vi "Launch Handler.vi"(7 "App Refnum":refnum<vi>, 8 "User action":bool=TRUE, 9 "Open":bool=TRUE, 10 "Diagram":bool=TRUE, 11 "VI":string) -> ()   [LabVIEW 2020, in "Peek Window.lvlib"]
uses:
  Peek Window.lvlib
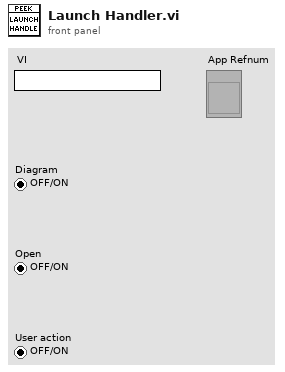
[diagram p1: front panel]
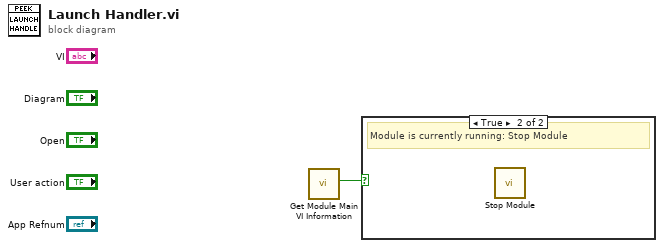
[diagram p0: block diagram]
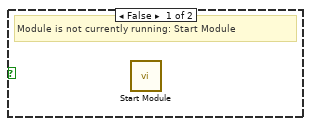
[diagram p2: hidden frame]
diagram:
  n1 = call "Get Module Main VI Information.vi"() -> ("Is Module Running?"=w1:bool)  [unwired: 8 in, 3 out]
  n2 = case shown="True" w1 {
    frame False {
      # "Module is not currently running: Start Module"
      n3 = call "Start Module.vi"() -> ()  [unwired: 8 in, 4 out]
    }
    frame True {
      # "Module is currently running: Stop Module"
      n4 = call "Stop Module.vi"() -> ()  [unwired: 11 in, 1 out]
    }
  }
